vi "Configure Execution View Manager.vi"(8 "error in (no error)":errorcluster, 11 "TS UI Data in":T1) -> (0 "error out":errorcluster, 3 "TS UI Data out":T1)   [LabVIEW 2015]
uses:
  Type defs/TS UI Data.ctl
  Type defs/Nest cluster.ctl
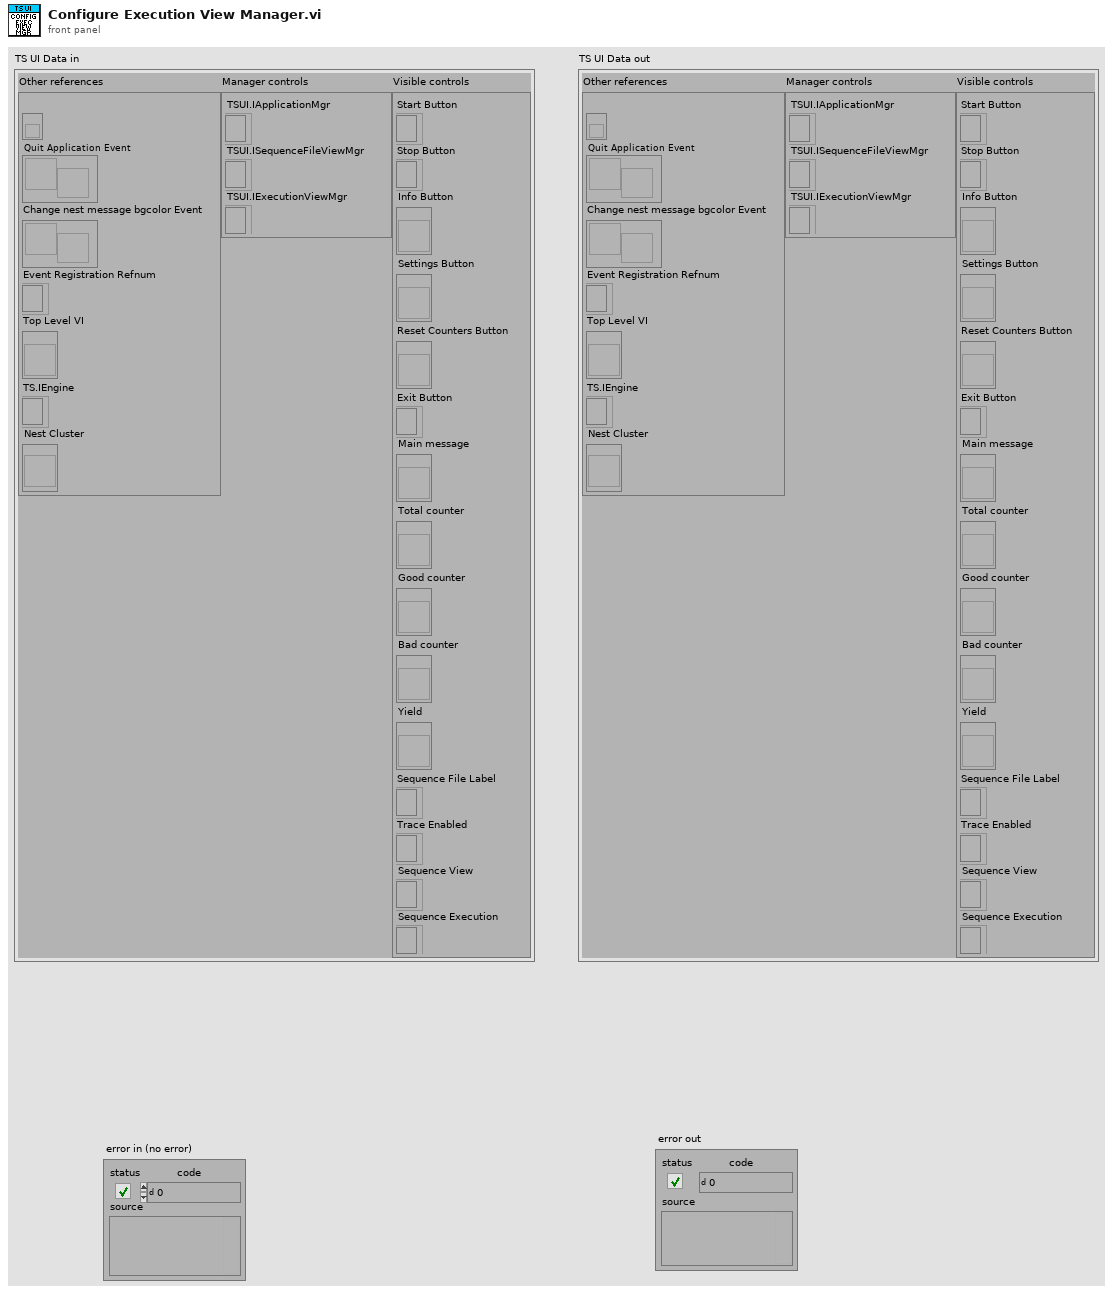
[diagram p1: front panel]
types:
  T1 = typedef "TS UI Data.ctl" = cluster{"Other references":cluster{"event callback refnum":refnum<k27>, "Quit Application Event":refnum<user-event>, "Change nest message bgcolor Event":refnum<user-event>, "event registration refnum":refnum<event-registration>, "Top Level VI":refnum<vi>, "TS.IEngine":refnum<k7>, "Nest Cluster":refnum<vi>}, "Manager controls":cluster{"TSUI.IApplicationMgr":refnum<k7>, "TSUI.ISequenceFileViewMgr":refnum<k7>, "TSUI.IExecutionViewMgr":refnum<k7>}, "Visible controls":cluster{"Start Button":refnum<k7>, "Stop Button":refnum<k7>, "Info Button":refnum<vi>, "Settings Button":refnum<vi>, "Reset Counters Button":refnum<vi>, "Exit Button":refnum<k7>, "Main message":refnum<vi>, "Total counter":refnum<vi>, "Good counter":refnum<vi>, "Bad counter":refnum<vi>, "Yield":refnum<vi>, "Sequence File Label":refnum<k7>, "Trace Enabled":refnum<k7>, "Sequence View":refnum<k7>, "Sequence Execution":refnum<k7>}}
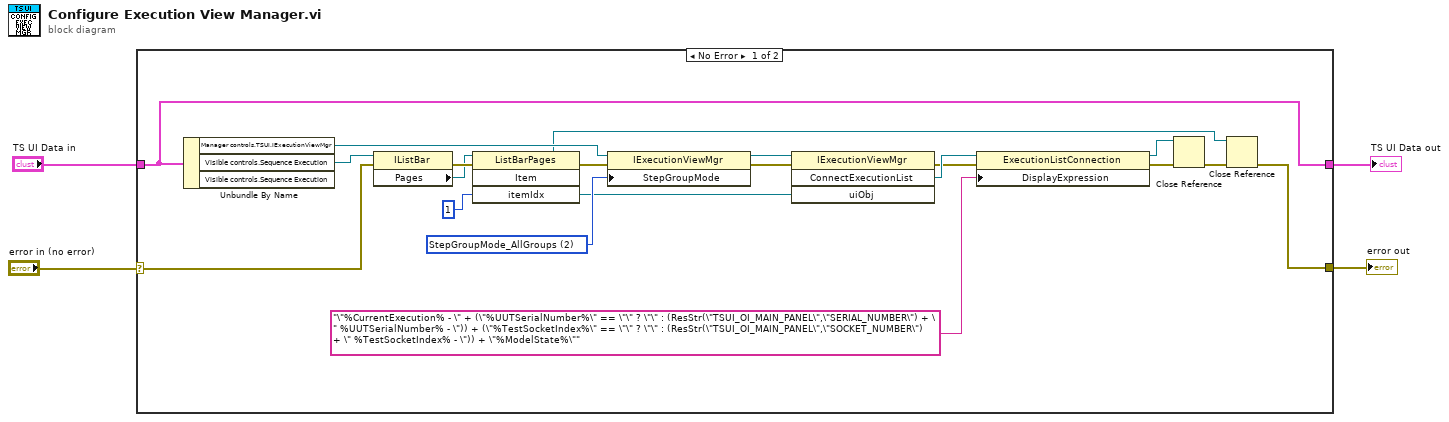
[diagram p0: block diagram]
diagram:
  n1 = case shown="No Error" "error in (no error)" {
    selector: "error in (no error)" -> [w22 w24]
    tunnel: "TS UI Data in" -> [w23 w25]
    tunnel: [w23 w25] -> w2
    tunnel: [w7 w24] -> w1
    frame No Error {
      w15 = 2 items=["StepGroupMode_OneGroup"=1, "StepGroupMode_AllGroups"=2] ("StepGroupMode")
      n2 = Unbundle By Name(w23) -> ("Manager controls.TSUI.IExecutionViewMgr"=w16:refnum<k7>, "Visible controls.Sequence Execution"=w21:refnum<k7>)  [unwired: 1 out]
      n3 = property class="IListBar"(reference=w21, error in=w22) -> (error out=w19:errorcluster, "Pages"=w18:refnum<k7>)  [unwired: 1 out]
      n4 = invoke class="ListBarPages" method="Item"(reference=w18, error in=w19, "itemIdx"=1) -> (error out=w17:errorcluster, "Item"=w6:refnum<k7>)  [unwired: 1 in, 2 out]
      n5 = property class="IExecutionViewMgr"(reference=w16, error in=w17, "StepGroupMode"=w15) -> (reference out=w14:refnum<k7>, error out=w13:errorcluster)
      n6 = invoke class="IExecutionViewMgr" method="ConnectExecutionList"(reference=w14, error in=w13, "uiObj"=w6) -> (error out=w5:errorcluster, "ConnectExecutionList"=w12:refnum<k7>)  [unwired: 1 in, 2 out]
      n7 = property class="ExecutionListConnection"(reference=w12, error in=w5, "DisplayExpression"="\"%CurrentExecution% - \" + (\"%UUTSerialNumber%\" == \"\" ? \"\" : (ResStr(\"TSUI_OI_MAIN_PANEL\",\"SERIAL_NUMBER\") + \" %UUTSerialNumber% - \")) + (\"%TestSocketIndex%\" == \"\" ? \"\" : (ResStr(\"TSUI_OI_MAIN_PANEL\",\"SOCKET_NUMBER\") + \" %TestSocketIndex% - \")) + \"%ModelState%\"") -> (reference out=w9:refnum<k7>, error out=w10:errorcluster)
      n8 = Close Reference(reference=w9, error in (no error)=w10) -> (error out=w8:errorcluster)
      n9 = Close Reference(reference=w6, error in (no error)=w8) -> (error out=w7:errorcluster)
    }
    frame Error {
    }
  }
  "TS UI Data out" <- w2
  "error out" <- w1
